vi "Create Scope Info Map for Each Site.vi"(8 "error in (no error)":errorcluster, 9 "parameters array":T1[](array[typedef]) {"reference position" format="%#_13g"; "min sample rate" format="%#_13p"; "maximum input frequency" format="%#_13p"; "input impedance" items=["1 mega ohm"=0, "50 ohms"=2]; "vertical coupling" items=["AC", "DC", "Ground"]; "probe attenuation" format="%.1f"; "vertical offset" format="%.4f"; "vertical range" format="%#_13g"}, 10 "Pin Names for Scope":string[](array[string]), 11 "connection map":map{string, T4[]}(c390)) -> (0 "error out":errorcluster, 3 "scope info map for each site":T3(array[numeric]))   [LabVIEW 2021, in "PMIC Common.lvlib"]
uses:
  PMIC Common.lvlib
  <instrlib>/niScope/Controls/niScope vertical coupling.ctl
  Scope Parameters.ctl
  Instrument Info.ctl
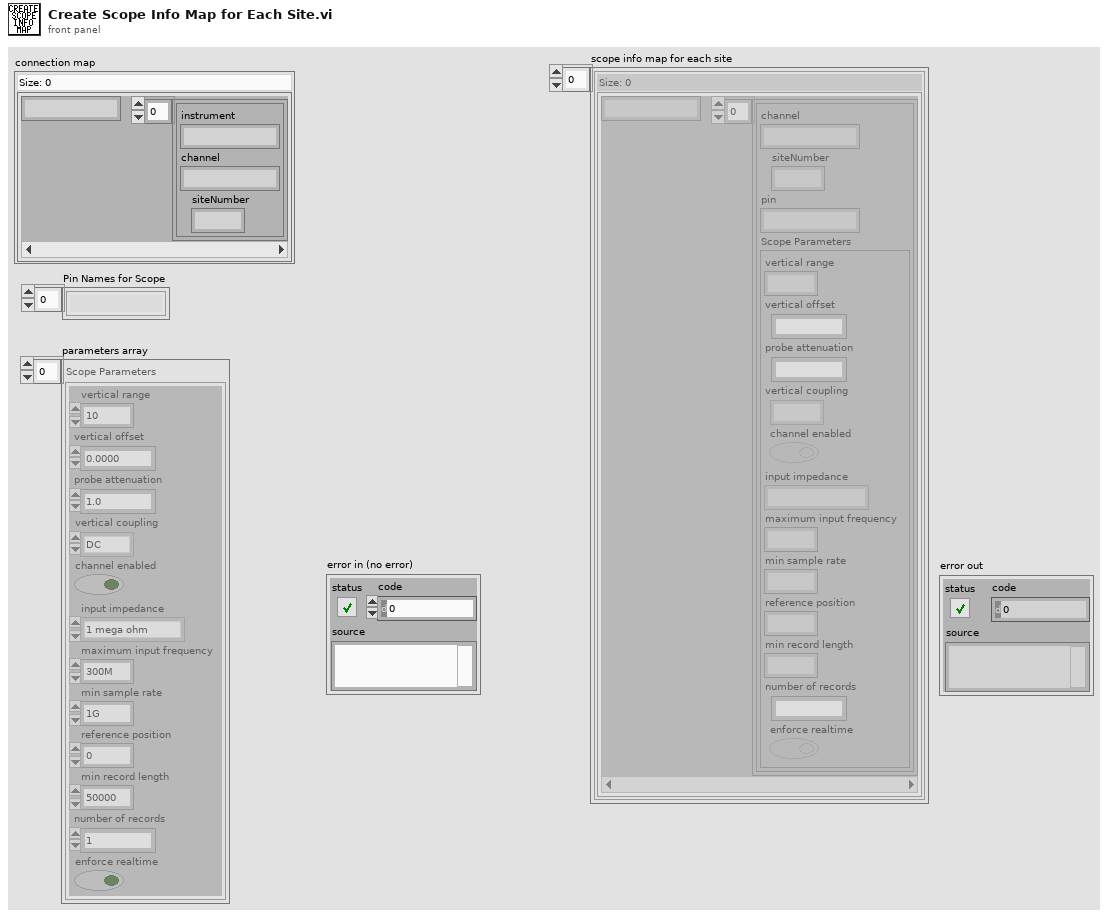
[diagram p1: front panel]
types:
  T1 = typedef "PMIC Common.lvlib/Scope Parameters.ctl" = cluster{"vertical range":dbl, "vertical offset":dbl, "probe attenuation":dbl, "vertical coupling":T2, "channel enabled":bool, "input impedance":u32, "maximum input frequency":dbl, "min sample rate":dbl, "reference position":dbl, "min record length":i32, "number of records":i32, "enforce realtime":bool}
  T2 = typedef "niScope vertical coupling.ctl" = i32
  T3 = map{string, cluster{"channel":string, "siteNumber":i32, "pin":string, "Scope Parameters":T1}[]}[]
  T4 = typedef "PMIC Common.lvlib/Instrument Info.ctl" = cluster{"instrument":string, "channel":string, "siteNumber":i32}
  T5 = map{string, cluster{"channel":string, "siteNumber":i32, "pin":string, "Scope Parameters":T1}[]}
  T6 = cluster{"channel":string, "siteNumber":i32, "pin":string, "Scope Parameters":T1}[]
  T7 = cluster{"channel":string, "siteNumber":i32, "String":string, "Scope Parameters":T1}
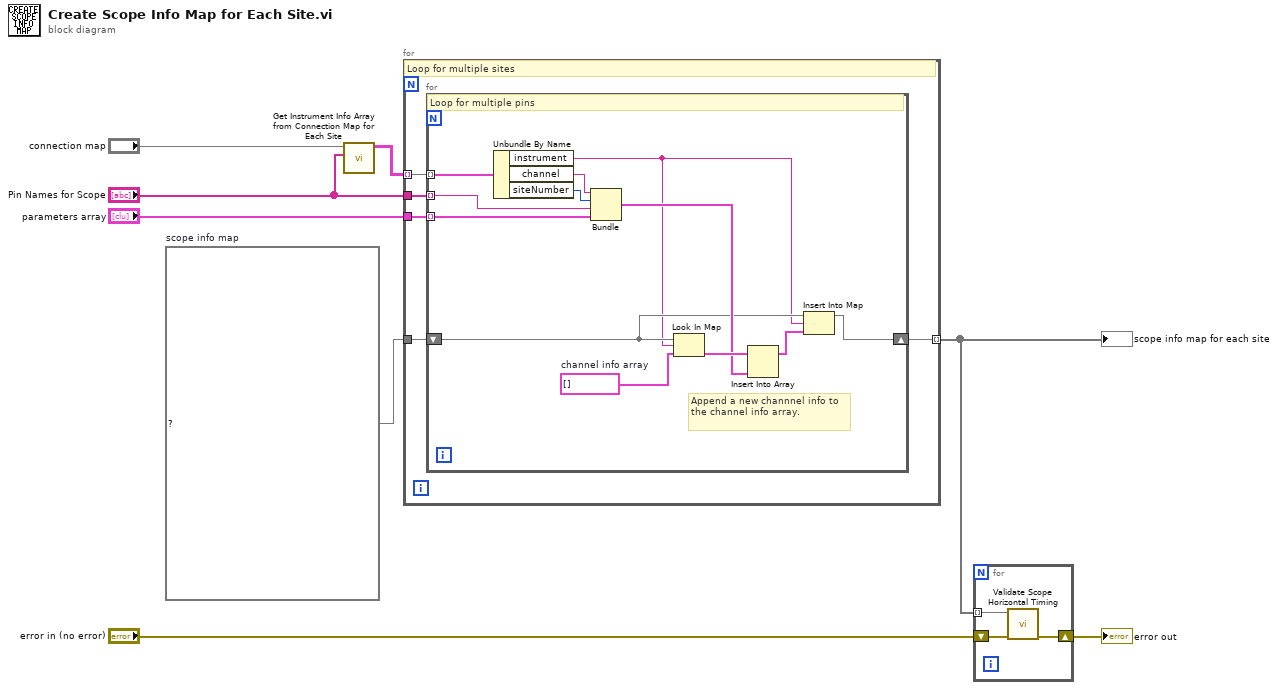
[diagram p0: block diagram]
diagram:
  w7 = T5 {}  # scope info map
  n1 = call "Get Instrument Info Array from Connection Map for Each Site.vi"("Pin Names for Scope"="Pin Names for Scope", "connection map"="connection map") -> ("instrument info array for each site"=w6:T4[][])  [unwired: 9 in]
  n2 = for {
    tunnel: w6 -> [w13] mode=indexing
    tunnel: "parameters array" -> [w12]
    tunnel: w7 -> [w11]
    tunnel: [w10] -> w3 mode=indexing
    tunnel: "Pin Names for Scope" -> [w9]
    # "Loop for multiple sites"
    n3 = for {
      tunnel: w13 -> [w24] mode=indexing
      tunnel: w12 -> [w15] mode=indexing
      shift-right: [w17] -> w10
      shift-left: w11 -> [w20]
      tunnel: w9 -> [w14] mode=indexing
      w16 = T6 []  # channel info array
      # "Append a new channnel info to the channel info array."
      # "Loop for multiple pins"
      n4 = Unbundle By Name(w24) -> ("instrument"=w18:string, "channel"=w25:string, "siteNumber"=w23:i32)
      n5 = Bundle("channel"=w25, "siteNumber"=w23, "String"=w14, "Scope Parameters"=w15) -> (w21:T7)  [unwired: 1 in]
      n6 = Look In Map(map=w20, key=w18, default value=w16) -> (value=w22:T6)  [unwired: 1 out]
      n7 = Insert Into Array(array=w22, new element=w21) -> (w19:T6)  [unwired: 1 in]
      n8 = Insert Into Map(map in=w20, key=w18, value=w19) -> (map out=w17:T5)  [unwired: 2 out]
    }
  }
  "scope info map for each site" <- w3
  n9 = for {
    tunnel: w3 -> [w28] mode=indexing
    shift-right: [w27] -> w1
    shift-left: "error in (no error)" -> [w26]
    n10 = call "Validate Scope Horizontal Timing.vi"("error in (no error)"=w26, "scope info map"=w28) -> ("error out"=w27:errorcluster)  [unwired: 9 in]
  }
  "error out" <- w1
